vi "KE2260B Read Internal Resistance.vi"(8 "error in (no error)":errorcluster, 11 "VISA resource name":refnum<visa-resource-name>) -> (0 "error out":errorcluster, 2 "Internal Resistance":dbl format="%.3g", 3 "VISA resource name out":refnum<visa-resource-name>)   [LabVIEW 2009, in "Keithley 2260B.lvlib"]
doc: "Returns the internal resistance of the power supply."
uses:
  <instrlib>/Keithley 2260B/Keithley 2260B.lvlib
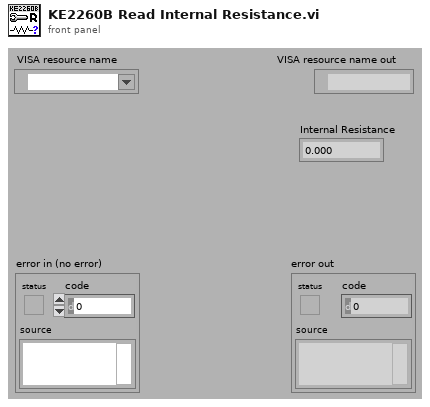
[diagram p1: front panel]
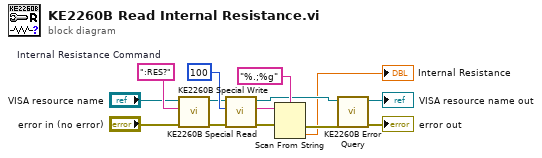
[diagram p0: block diagram]
diagram:
  w7 = ":RES?"  # Internal Resistance Command
  n1 = call <instrlib>:"KE2260B Special Write.vi"("error in (no error)"="error in (no error)", "Write Buffer (\"\")"=w7, "VISA session"="VISA resource name") -> ("error out"=w9:errorcluster, "dup VISA session"=w8:refnum<visa-resource-name>)  [unwired: 6 in, 1 out]
  n2 = call <instrlib>:"KE2260B Special Read.vi"("error in (no error)"=w9, "byte count"=u32 100, "VISA session"=w8) -> ("error out"=w4:errorcluster, "read buffer"=w11:string, "dup VISA session"=w3:refnum<visa-resource-name>)  [unwired: 5 in, 1 out]
  n3 = Scan From String(format string="%.;%g", input string=w11, error in=w4) -> (error out=w2:errorcluster, output 1=→"Internal Resistance":dbl)  [unwired: 2 in, 2 out]
  n4 = call <instrlib>:"KE2260B Error Query.vi"("error in (no error)"=w2, "VISA resource name"=w3) -> ("error out"=→"error out":errorcluster, "VISA resource name out"=→"VISA resource name out":refnum<visa-resource-name>)  [unwired: 6 in, 2 out]
